vi "Scale_stable_weight.vi"(4 "error in (no error)":errorcluster, 7 "VISA resource name":refnum<visa-resource-name>) -> (0 "error out":errorcluster, 1 "Number after conversion":dbl, 2 "read buffer":string, 3 "VISA resource name out":refnum<visa-resource-name>)   [LabVIEW 2019]
panel:
  out "Number before conversion":string
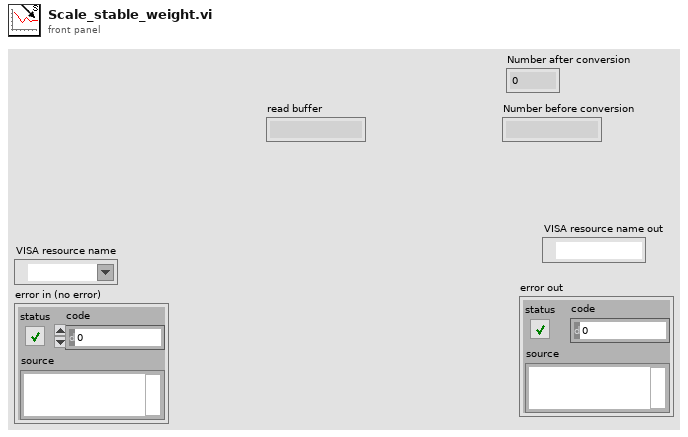
[diagram p1: front panel]
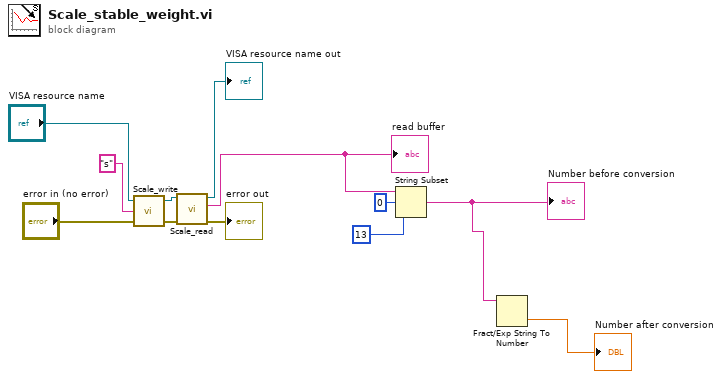
[diagram p0: block diagram]
diagram:
  n1 = call "Scale_write.vi"("error in (no error)"="error in (no error)", "write buffer"="s", "VISA resource name"="VISA resource name") -> ("error out"=w8:errorcluster, "VISA resource name out"=w9:refnum<visa-resource-name>)  [unwired: 1 in]
  n2 = call "Scale_read.vi"("error in (no error)"=w8, "VISA resource name"=w9) -> ("error out"=→"error out":errorcluster, "read buffer"=w5:string, "VISA resource name out"=→"VISA resource name out":refnum<visa-resource-name>)  [unwired: 2 in, 1 out]
  "read buffer" <- w5
  n3 = String Subset(string=w5, offset (0)=0, length (rest)=13 ("length (rest)")) -> (substring=w2:string)
  "Number before conversion" <- w2
  n4 = Fract/Exp String To Number(string=w2) -> (number=→"Number after conversion":dbl)  [unwired: 3 in, 1 out]
